vi "Remove_Spikes_Low.vi"(3 "index":i32, 4 "Background noise":dbl, 5 "Time Trace":dbl[](graph)) -> (0 "Spike":bool, 1 "Filtered Time Trace":dbl[](graph))   [LabVIEW 2011]
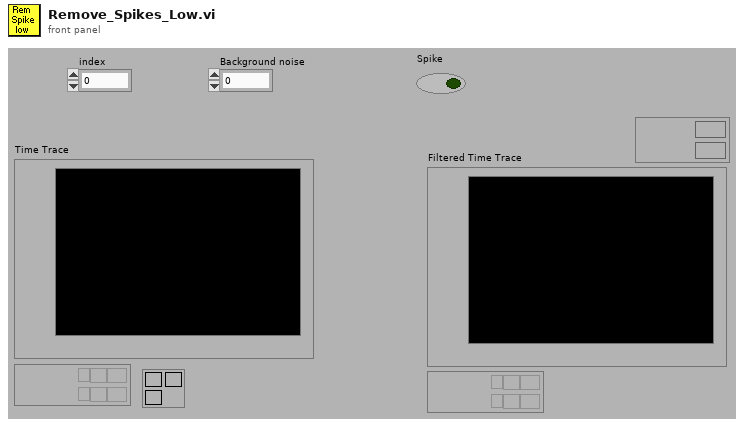
[diagram p1: front panel]
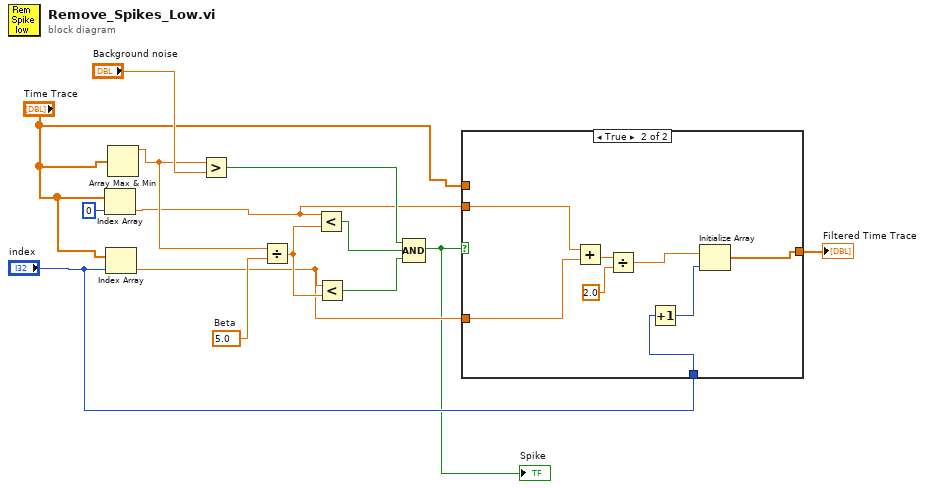
[diagram p0: block diagram]
diagram:
  w11 = 5.0  # Beta
  n1 = Index Array(array="Time Trace", index=0) -> (element=w4:dbl)
  n2 = Index Array(array="Time Trace", index="index") -> (element=w3:dbl)
  n3 = Array Max & Min(array="Time Trace") -> (max value=w12:dbl)  [unwired: 3 out]
  n4 = Greater?(x=w12, y="Background noise") -> (0:w9:bool)
  n5 = Divide(x=w12, y=w11) -> (x/y=w10:dbl)
  n6 = Less?(x=w4, y=w10) -> (x < y?=w8:bool)
  n7 = Less?(x=w3, y=w10) -> (x < y?=w7:bool)
  n8 = Compound Arithmetic op=AND(w9, w8, w7) -> (w1:bool)
  "Spike" <- w1
  n9 = case shown="True" w1 {
    tunnel: [w15 w16] -> w6
    tunnel: "Time Trace" -> [w15 _]
    tunnel: w4 -> [_ w23]
    tunnel: w3 -> [_ w22]
    tunnel: "index" -> [_ w18]
    frame False {
    }
    frame True {
      n10 = Add(x=w23, y=w22) -> (x+y=w21:dbl)
      n11 = Divide(x=w21, y=2.0) -> (x/y=w19:dbl)
      n12 = Increment(x=w18) -> (x+1=w17:i32)
      n13 = Initialize Array(w19, w17) -> (w16:dbl[])
    }
  }
  "Filtered Time Trace" <- w6
